vi "Read Configuration Data.vi"(8 "error in (no error)":errorcluster caption="entrée d'erreur (pas d'erreur)") -> (0 "error out":errorcluster caption="sortie d'erreur", 3 "Configuration data":T1)   [LabVIEW 2013, in "Data Configuration File.lvlib"]
doc: "Ce VI lit le fichier de configuration et rend sous forme de cluster les données d'initialisation"
uses:
  Data Configuration File.lvlib
  Data Config.ctl
  <vilib>/Utility/config.llb/NI_LVConfig.lvlib
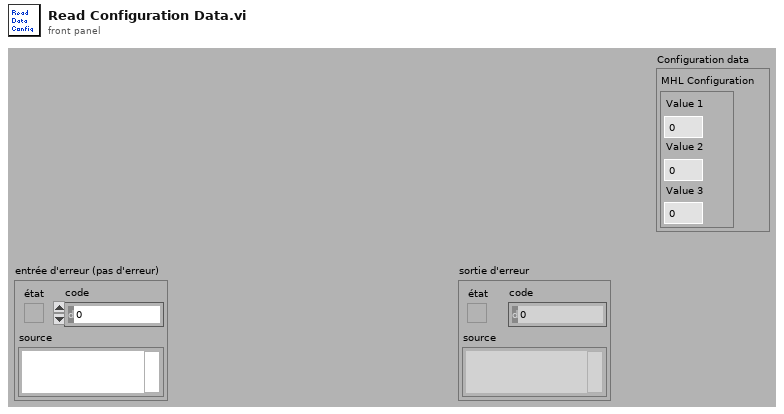
[diagram p1: front panel]
types:
  T1 = typedef "Data Configuration File.lvlib/Data Config.ctl" = cluster{"MHL Configuration":cluster{"Value 1":dbl, "Value 2":dbl, "Value 3":dbl}}
  T2 = enum32{"invalid app kind", "Development System", "Run Time System", "Student Edition", "Embedded LabVIEW", "Evaluation", "Custom"}
  T3 = typedef "NI_LVConfig.lvlib/Config Data RefNum.ctl" = refnum<k1>
  T4 = typedef "Data Configuration File.lvlib/MHL configuration.ctl" = cluster{"Value 1":dbl, "Value 2":dbl, "Value 3":dbl}
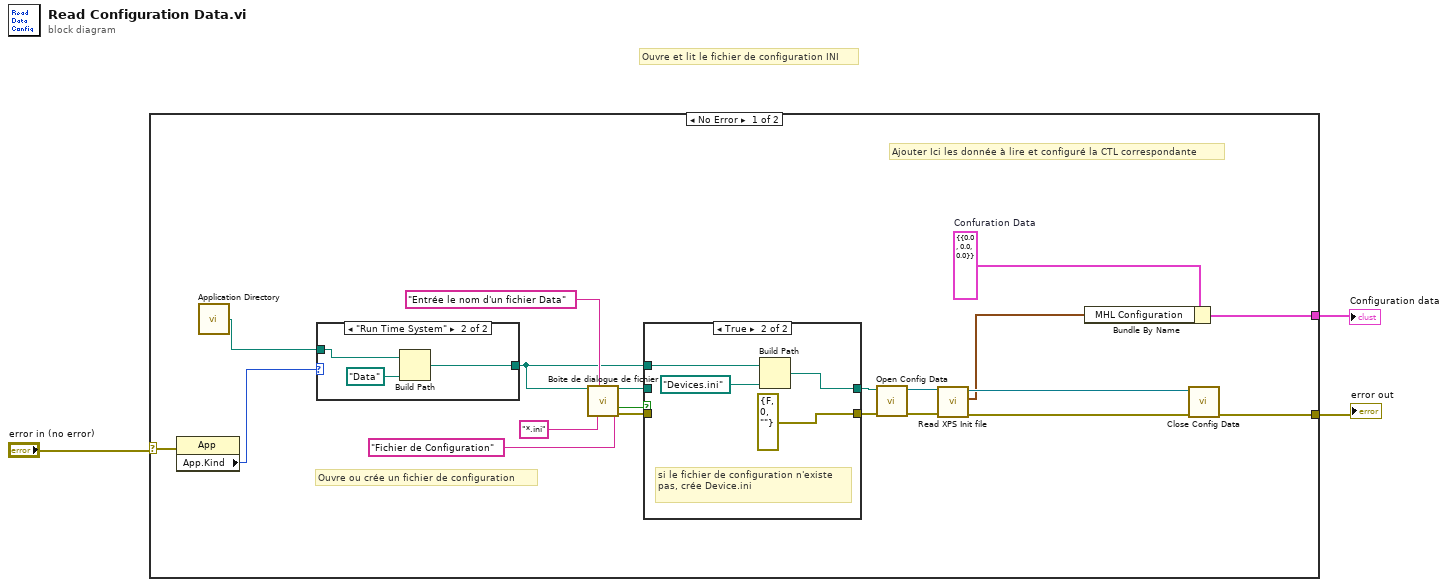
[diagram p0: block diagram]
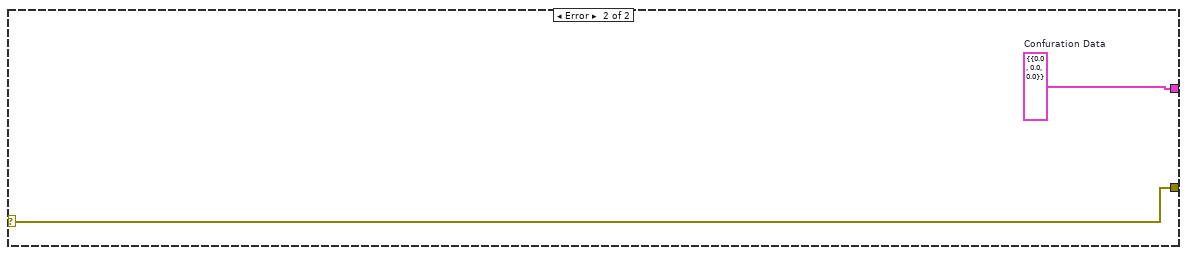
[diagram p4: hidden frame]
diagram:
  # "Ouvre et lit le fichier de configuration INI"
  n1 = case shown="No Error" "error in (no error)" {
    selector: "error in (no error)" -> [w23 w35]
    tunnel: [w13 w35] -> w2
    tunnel: [w5 w34] -> w1
    frame No Error {
      w6 = T1 {"MHL Configuration"={"Value 1"=0.0, "Value 2"=0.0, "Value 3"=0.0}}  # Confuration Data
      # "Ajouter Ici les donnée à lire et configuré la CTL correspondante"
      # "Ouvre ou crée un fichier de configuration"
      n2 = property class="App"(error in=w23) -> ("App.Kind"=w22:T2)  [unwired: 1 in, 2 out]
      n3 = call <vilib>:"Application Directory.vi"() -> ("Application Directory"=w11:path)
      n4 = case shown="\"Run Time System\"" w22 {
        tunnel: w11 -> [w30 w33]
        tunnel: [w30 w31] -> w12
        frame Default {
        }
        frame "Run Time System" {
          n5 = Build Path(base path=w33, name or relative path=path "Data") -> (appended path=w31:path)
        }
      }
      n6 = call "Boîte de dialogue de fichier"("start path"=w12, "prompt"="Entrée le nom d'un fichier Data", "pattern (all files)"="*.ini", "pattern label"="Fichier de Configuration") -> ("selected path"=w16:path, "cancelled"=w18:bool, "error out"=w17:errorcluster)  [unwired: 8 in, 1 out]
      n7 = case shown="True" w18 {
        tunnel: w12 -> [_ w29]
        tunnel: [w25 errorcluster {"status"=FALSE, "code"=0, "source"=""} ("error in (no error)")] -> w15
        tunnel: [w24 w26] -> w14
        tunnel: w17 -> [w25 _]
        tunnel: w16 -> [w24 _]
        frame False {
        }
        frame True {
          # "si le fichier de configuration n'existe pas, crée Device.ini"
          n8 = Build Path(base path=w29, name or relative path=path "Devices.ini") -> (appended path=w26:path)
        }
      }
      n9 = call <vilib>:"Open Config Data.vi"("error in (no error)"=w15, "configuration file path"=w14) -> ("error out"=w10:errorcluster, "refnum"=w9:T3)  [unwired: 7 in, 1 out]
      n10 = call "Read XPS Init file.vi"("error in"=w10, "refnum in"=w9) -> ("error out"=w8:errorcluster, "MHL Configuration"=w4:T4, "refnum out"=w7:T3)  [unwired: 7 in]
      n11 = Bundle By Name(cluster=w6, "MHL Configuration"=w4) -> (w5:T1)
      n12 = call <vilib>:"Close Config Data.vi"("error in (no error)"=w8, "refnum"=w7) -> ("error out"=w13:errorcluster)  [unwired: 8 in, 1 out]
    }
    frame Error {
      w34 = T1 {"MHL Configuration"={"Value 1"=0.0, "Value 2"=0.0, "Value 3"=0.0}}  # Confuration Data
    }
  }
  "error out" <- w2
  "Configuration data" <- w1
